vi "PID (SubVI).vi"(0 "Sample time (ms)":dbl, 2 "Set Point":dbl, 4 "upper limit":dbl, 5 "Reset PID":bool, 6 "lower limit":dbl, 7 "Kp":dbl, 9 "Ki":dbl, 11 "Kd":dbl, 12 "Process Value":dbl) -> (15 "PID out":dbl)   [LabVIEW 2019]
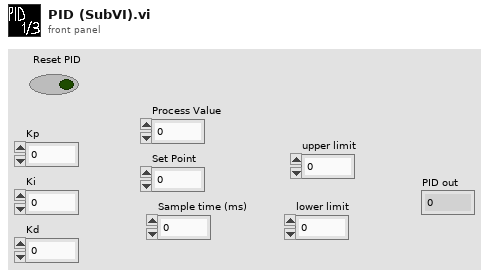
[diagram p1: front panel]
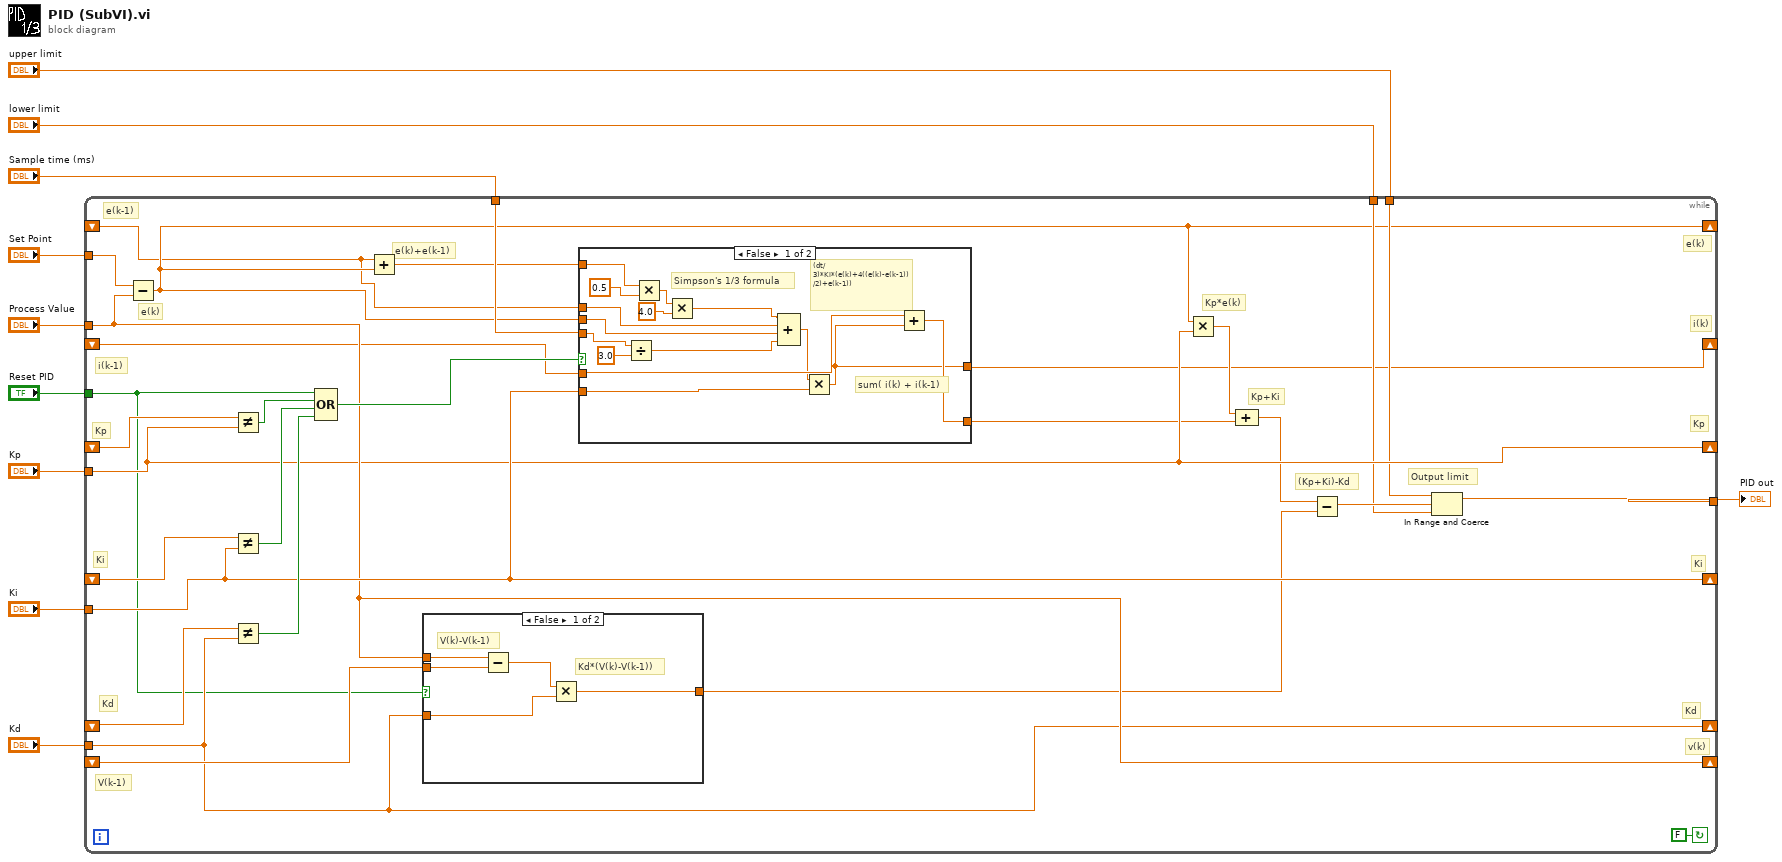
[diagram p0: block diagram]
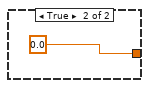
[diagram p2: hidden frame]
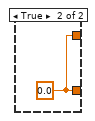
[diagram p3: hidden frame]
diagram:
  n1 = while {
    shift-right: [w16] -> _
    shift-left: _ -> [w15]
    tunnel: "Reset PID" -> [w22]
    tunnel: "Set Point" -> [w32]
    tunnel: "Kd" -> [w27]
    tunnel: "Ki" -> [w31]
    tunnel: "Kp" -> [w23]
    shift-right: [w23] -> _
    shift-left: _ -> [w33]
    shift-right: [w31] -> _
    shift-left: _ -> [w34]
    shift-right: [w27] -> _
    shift-left: _ -> [w35]
    tunnel: "Process Value" -> [w29]
    shift-right: [w12] -> _
    shift-left: _ -> [w17]
    shift-right: [w29] -> _
    shift-left: _ -> [w28]
    tunnel: "Sample time (ms)" -> [w30]
    tunnel: "lower limit" -> [w20]
    tunnel: "upper limit" -> [w19]
    tunnel: [w25] -> w2
    stop <- FALSE continue-if-true
    # "i(k)"
    # "(Kp+Ki)-Kd"
    # "Kp+Ki"
    # "Output limit"
    # "e(k)+e(k-1)"
    # "e(k)"
    # "Kp*e(k)"
    # "v(k)"
    # "Kd"
    # "Ki"
    # "e(k)"
    # "Kp"
    # "Kp"
    # "Kd"
    # "Ki"
    # "i(k-1)"
    # "V(k-1)"
    # "e(k-1)"
    n2 = Subtract(x=w32, y=w29) -> (x-y=w16:dbl)
    n3 = Not Equal?(x=w33, y=w23) -> (x != y?=w11:bool)
    n4 = Not Equal?(x=w34, y=w31) -> (x != y?=w37:bool)
    n5 = Not Equal?(x=w35, y=w27) -> (x != y?=w36:bool)
    n6 = Compound Arithmetic op=OR(w22, w11, w37, w36) -> (w38:bool)
    n7 = Add(x=w15, y=w16) -> (x+y=w24:dbl)
    n8 = case shown="False" w22 {
      tunnel: w29 -> [w44 _]
      tunnel: w28 -> [w43 _]
      tunnel: w27 -> [w41 _]
      tunnel: [w40 0.0] -> w14
      frame False {
        # "Kd*(V(k)-V(k-1))"
        # "V(k)-V(k-1)"
        n9 = Subtract(x=w44, y=w43) -> (x-y=w42:dbl)
        n10 = Multiply(x=w42, y=w41) -> (x*y=w40:dbl)
      }
      frame True {
      }
    }
    n11 = case shown="False" w38 {
      tunnel: [w60 w61] -> w13
      tunnel: w31 -> [w59 _]
      tunnel: w30 -> [w55 _]
      tunnel: w17 -> [w58 _]
      tunnel: w24 -> [w53 _]
      tunnel: w16 -> [w48 _]
      tunnel: w15 -> [w47 _]
      tunnel: [w46 w61] -> w12
      frame False {
        # "Simpson's 1/3 formula"
        # "sum( i(k) + i(k-1)"
        # "(dt/3)*Ki*(e(k)+4((e(k)-e(k-1))/2)+e(k-1))"
        n12 = Divide(x=w55, y=3.0) -> (x/y=w54:dbl)
        n13 = Multiply(x=w53, y=0.5) -> (x*y=w50:dbl)
        n14 = Multiply(x=w50, y=4.0) -> (x*y=w49:dbl)
        n15 = Compound Arithmetic op=ADD(w49, w47, w48, w54) -> (w57:dbl)
        n16 = Multiply(x=w57, y=w59) -> (x*y=w46:dbl)
        n17 = Add(x=w58, y=w46) -> (x+y=w60:dbl)
      }
      frame True {
        w61 = 0.0
      }
    }
    n18 = Multiply(x=w16, y=w23) -> (x*y=w18:dbl)
    n19 = Compound Arithmetic op=ADD(w18, w13) -> (w21:dbl)
    n20 = Subtract(x=w21, y=w14) -> (x-y=w26:dbl)
    n21 = In Range and Coerce(upper limit=w19, x=w26, lower limit=w20) -> (coerced(x)=w25:dbl)  [unwired: 1 out]
  }
  "PID out" <- w2
